vi "CS-4 Utility Default Instrument Setup.vi"(8 "error in (no error)":errorcluster, 11 "VISA session":refnum<visa-resource-name>) -> (0 "error out":errorcluster, 3 "dup VISA session":refnum<visa-resource-name>)   [LabVIEW 2016]
doc: "This Utility VI sends a default command string to the instrument whenever a new VISA session is opened, or the instrument is reset. This VI is intended to be used as a subVI for the CS-4 Initialize and CS-4 Reset VI's. Altering this VI could cause these two VI's to operate incorrectly."
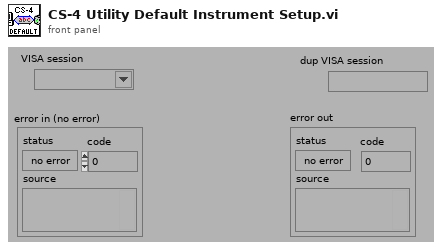
[diagram p1: front panel]
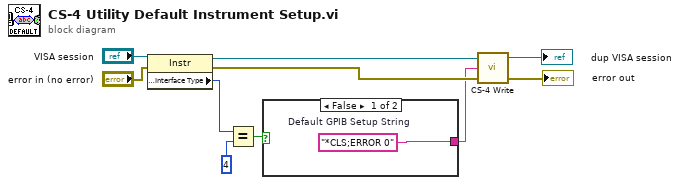
[diagram p0: block diagram]
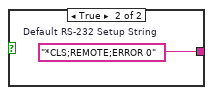
[diagram p2: hidden frame]
diagram:
  n1 = property class="Instr"(reference="VISA session", error in="error in (no error)") -> (reference out=w3:refnum<visa-resource-name>, error out=w2:errorcluster, "Interface Information:Interface Type"=w5:u16)
  n2 = Equal?(x=w5, y=u16 4) -> (x = y?=w7:bool)
  n3 = case shown="False" w7 {
    tunnel: [w11 w12] -> w1
    frame False {
      w11 = "*CLS;ERROR 0"  # Default GPIB Setup String
    }
    frame True {
      w12 = "*CLS;REMOTE;ERROR 0"  # Default RS-232 Setup String
    }
  }
  n4 = call "CS-4 Write.vi"("error in (no error)"=w2, "write buffer (\"\")"=w1, "VISA session"=w3) -> ("error out"=→"error out":errorcluster, "dup VISA session"=→"dup VISA session":refnum<visa-resource-name>)  [unwired: 1 out]
